vi "tcsOfc_acceptCommand_readWfsFile.vi"(8 "error in (no error)":errorcluster, 11 "command_readWfsFile_Ctl":T1={"fileName"="", "sensorIdList[189]"=[0, 0, 0, 0, 0, 0, 0, 0, 0, 0, 0, 0, 0, 0, 0, 0, 0, 0, 0, 0, 0, 0, 0, 0, 0, 0, 0, 0, 0, 0, 0, 0, 0, 0, 0, 0, 0, 0, 0, 0, 0, 0, 0, 0, 0, 0, 0, 0, 0, 0, 0, 0, 0, 0, 0, 0, 0, 0, 0, 0, 0, 0, 0, 0, 0, 0, 0, 0, 0, 0, 0, 0, 0, 0, 0, 0, 0, 0, 0, 0, 0, 0, 0, 0, 0, 0, 0, 0, 0, 0, 0, 0, 0, 0, 0, 0, 0, 0, 0, 0, 0, 0, 0, 0, 0, 0, 0, 0, 0, 0, 0, 0, 0, 0, 0, 0, 0, 0, 0, 0, 0, 0, 0, 0, 0, 0, 0, 0, 0, 0, 0, 0, 0, 0, 0, 0, 0, 0, 0, 0, 0, 0, 0, 0, 0, 0, 0, 0, 0, 0, 0, 0, 0, 0, 0, 0, 0, 0, 0, 0, 0, 0, 0, 0, 0, 0, 0, 0, 0, 0, 0, 0, 0, 0, 0, 0, 0, 0, 0, 0, 0, 0, 0, 0, 0, 0, 0, 0, 0]}) -> (0 "error out":errorcluster, 2 "function return":i32, 3 "command_readWfsFile_Ctl out":T1)   [LabVIEW 2016, in "SALLV_tcsOfc.lvlib"]
doc: "int tcsOfc_shm_acceptCommand_readWfsFileLV(tcsOfc_command_readWfsFileLV *command_readWfsFile_Ctl );"
uses:
  SALLV_tcsOfc.lvlib
  DataTypes/command_readWfsFile.ctl
  SALLV_tcsOfc.so
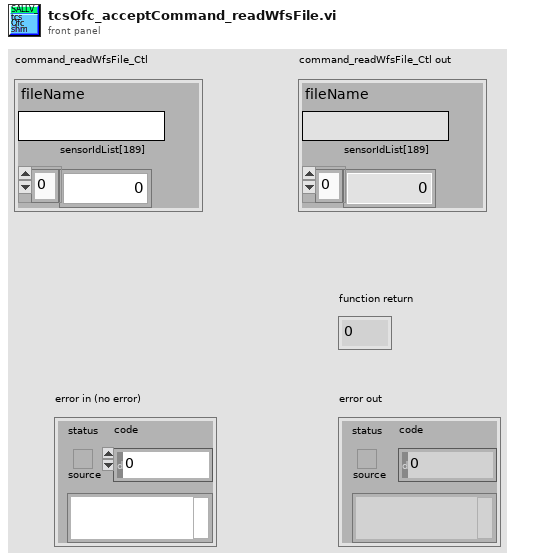
[diagram p1: front panel]
types:
  T1 = typedef "SALLV_tcsOfc.lvlib/command_readWfsFile.ctl" = cluster{"fileName":string, "sensorIdList[189]":i16[]}
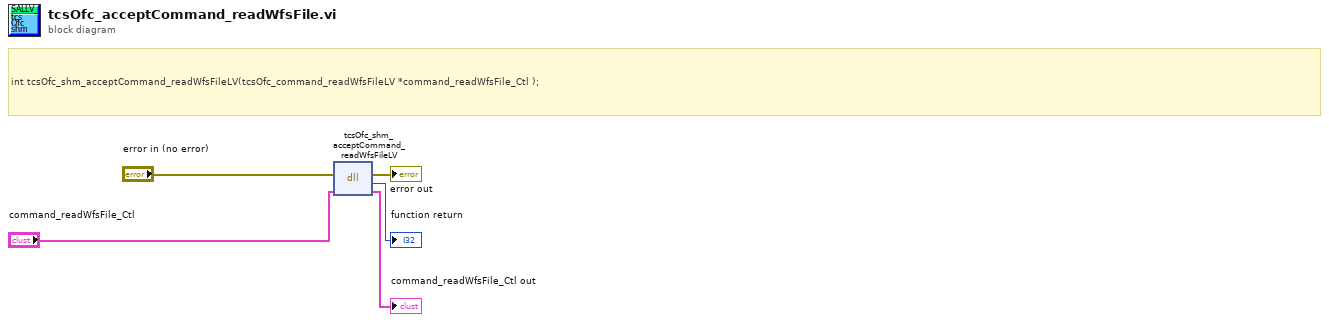
[diagram p0: block diagram]
diagram:
  # "int tcsOfc_shm_acceptCommand_readWfsFileLV(tcsOfc_command_readWfsFileLV *command_readWfsFile_Ctl );"
  n1 = dll-call lib="home/ttsai/Documents/salAPI/SALLV_tcsOfc/SALLV_tcsOfc.*" fn="tcsOfc_shm_acceptCommand_readWfsFileLV"(error in="error in (no error)", "command_readWfsFile_Ctl"="command_readWfsFile_Ctl") -> (error out=→"error out":errorcluster, →"function return":i32, "command_readWfsFile_Ctl"=→"command_readWfsFile_Ctl out":T1)  [unwired: 2 in, 1 out]
